vi "Send Command LB.vi"(8 "error in (no error)":errorcluster, 10 "output LB Command cluster":T1, 11 "TCP Network Connection in":refnum<k5>) -> (0 "error out":errorcluster)   [LabVIEW 2011]
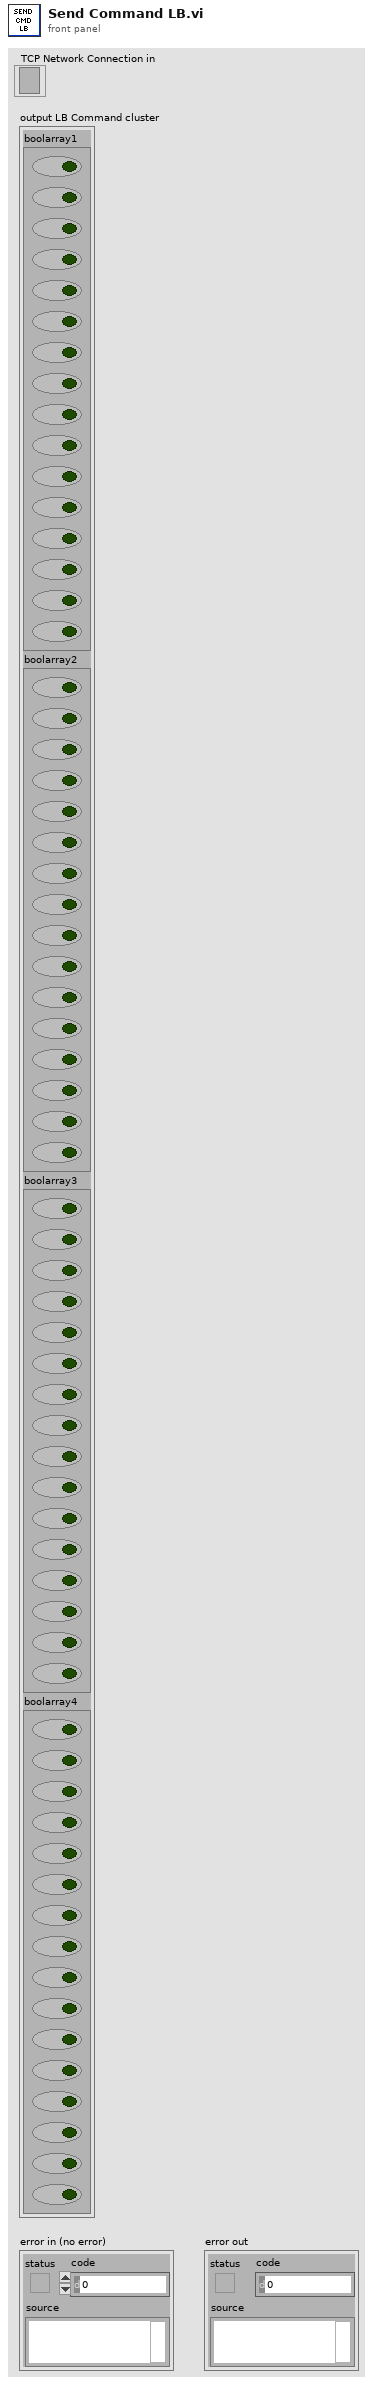
[diagram p1: front panel]
types:
  T1 = cluster{"boolarray1":cluster{bool, bool, bool, bool, bool, bool, bool, bool, bool, bool, bool, bool, bool, bool, bool, bool}, "boolarray2":cluster{bool, bool, bool, bool, bool, bool, bool, bool, bool, bool, bool, bool, bool, bool, bool, bool}, "boolarray3":cluster{bool, bool, bool, bool, bool, bool, bool, bool, bool, bool, bool, bool, bool, bool, bool, bool}, "boolarray4":cluster{bool, bool, bool, bool, bool, bool, bool, bool, bool, bool, bool, bool, bool, bool, bool, bool}}
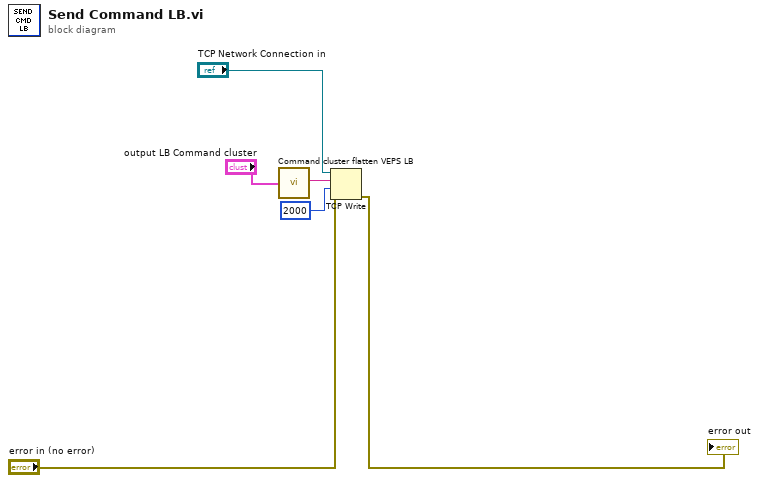
[diagram p0: block diagram]
diagram:
  n1 = call "Command cluster flatten VEPS LB.vi"("command"="output LB Command cluster") -> ("data string"=w2:string)  [unwired: 1 out]
  n2 = TCP Write(connection ID="TCP Network Connection in", data in=w2, error in (no error)="error in (no error)", 9:2000 ("ms timeout (10000)")) -> (error out=→"error out":errorcluster)  [unwired: 2 out]
